vi "rename to VIPT.vi"() -> (0 "error out":errorcluster)   [LabVIEW 2019]
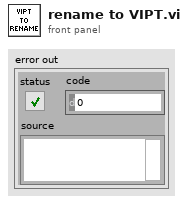
[diagram p1: front panel]
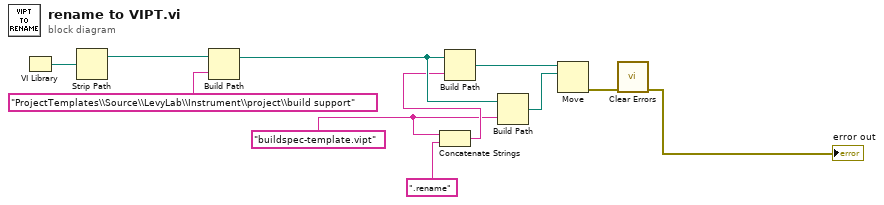
[diagram p0: block diagram]
diagram:
  w4 = "buildspec-template.vipt" ("name or relative path")
  n1 = VI Library() -> (path=w3:path)
  n2 = Strip Path(path=w3) -> (stripped path=w2:path)  [unwired: 1 out]
  n3 = Build Path(base path=w2, name or relative path="ProjectTemplates\\Source\\LevyLab\\Instrument\\project\\build support") -> (appended path=w9:path)
  n4 = Concatenate Strings(w4, ".rename" ("name or relative path")) -> (w5:string)
  n5 = Build Path(base path=w9, name or relative path=w5) -> (appended path=w10:path)
  n6 = Build Path(base path=w9, name or relative path=w4) -> (appended path=w8:path)
  n7 = Move(source path=w10, 10:w8) -> (error out=w7:errorcluster)  [unwired: 3 in, 2 out]
  n8 = call <vilib>:"Clear Errors.vi"("error in (no error)"=w7) -> ("error out"=→"error out":errorcluster)  [unwired: 5 in, 1 out]
